vi "AOIParams.vi"() -> ()   [LabVIEW 2022 SP3]
uses:
  <vilib>/Utility/file.llb/Read Delimited Spreadsheet (DBL).vi
  <vilib>/Analysis/NI_AALBase.lvlib
panel:
  in  "Range Params":T1={"mb max"=-20.0, "mb min"=-70.0, "slope max"=8.0, "slope min"=-8.0, "int max"=5.0, "int min"=-85.0} {"int min" format="%.2f"; "int max" format="%.2f"; "slope min" format="%.2f"; "slope max" format="%.2f"; "mb min" format="%.2f"; "mb max" format="%.2f"}
  in  "data type":u16(ring)=1 items=["Spreadsheet", "byte file"]
  in  "Save to params.txt?":bool
  in  "Log scaling?":bool=TRUE
  out "mean of\nintercept":dbl format="%.3f"
  out "mean of\nslope":dbl format="%.3f"
  in  "Data for AOI":u16(ring)=2 items=["MidBand Fit Ellipse", "MidBand Fit Draw", "MidBand Fit Rect", "Slope Ellipse", "Slope Draw", "Slope Rect", "Intercept Ellipse", "Intercept Draw", "Intercept Rect"]
  out "RF Info":T2
  out "Array slope":dbl[][](array[numeric]) format="%.2f"
  out "Array midband":dbl[][](array[numeric]) format="%.2f"
  out "mean of\nmidband fit":dbl format="%.3f"
  in  "Use AOI":bool
  out "Array intercept":dbl[][](array[numeric]) format="%.2f"
  in  "Rotation":u32(knob) scale=0.18..180.0
  out "sector image":dbl[][](graph)
  out "raw eye data":i16[][](graph)
  out "Fit Param Image":dbl[][](graph)
  out "Fit band":T3 {"center freq" format="%.2f"; "stop freq" format="%.2f"; "start" format="%.2f"}
  in  "new eye file path":path
  # "Choose original eye file to run program. Parameter files must be in a sub-folder of the eye files named Param Images."
  # "© 2000 Riverside Research Institute"
  # "For ellipse use all three cursors, yellow is center. For free draw mode, yellow cursor will trace out aea. Start and stop free draw by pressing F1 key.For rectrangular mode, yellow and green form box. Yellow must be above and to left of green."
  # "(Ignore if Fit Param Image already in sector form)"
  # "Only needed for byte files"
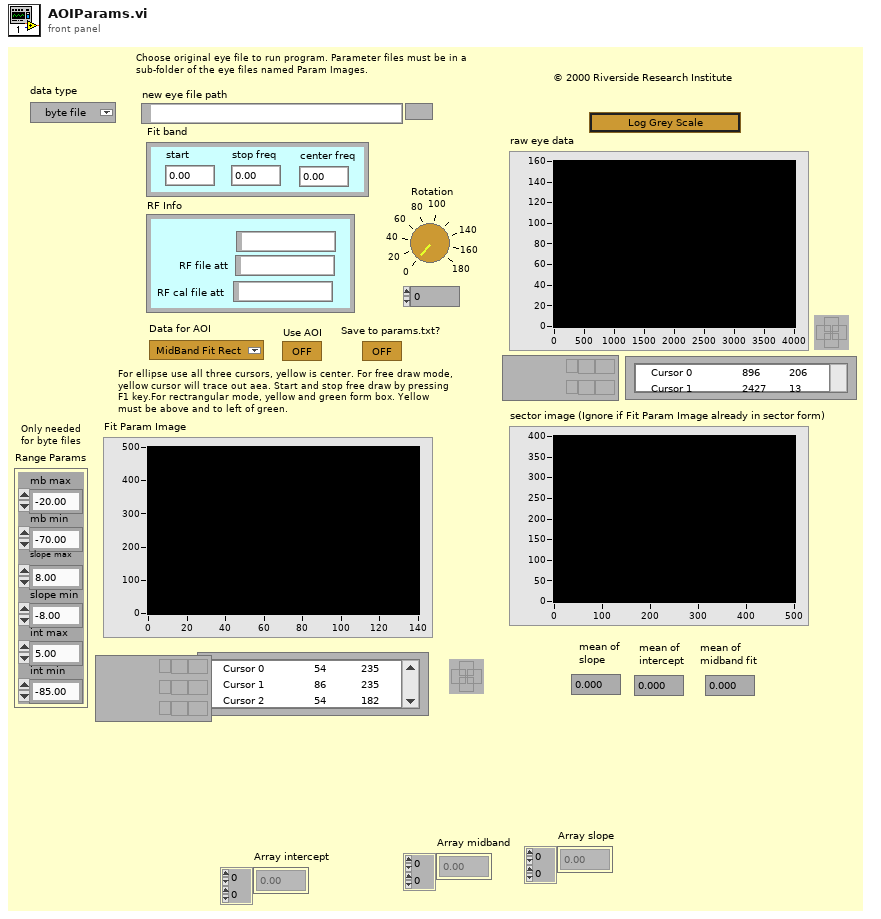
[diagram p1: front panel]
types:
  T1 = cluster{"mb max":dbl, "mb min":dbl, "slope max":dbl, "slope min":dbl, "int max":dbl, "int min":dbl}
  T2 = cluster{"RF file name":string, "RF file att":string, "RF cal file name":string, "RF cal file att":string}
  T3 = cluster{"start":dbl, "stop freq":dbl, "center freq":dbl}
  T4 = typedef "LVPointDoubleTypeDef.ctl" = cluster{"Cursor X":dbl, "Cursor Y":dbl}
  T5 = typedef "Header.ctl" = cluster{"header info":cluster{"Header":string, "Head length":i16}, "A/D info":cluster{"# rf points per line":u16, "# lines per scan":u16, "sample rate MHz":u16, "# A/D bits":i16, "# bytes per A/D":u16, "TGC Flag":u16, "A/D Type":string}, "Tranducer Info":cluster{"bandwidth":sgl, "center freq":sgl, "start freq":sgl, "ID":i32}, "Scan Info":cluster{"delay":sgl, "pivot distance":sgl, "sector scan angle":sgl, "operator":string, "Scan Mode":string, "location":string}, "Time/Date Info":cluster{"date":string, "time":string}, "RF Info":cluster{"RF file name":string, "RF file att":string, "RF cal file name":string, "RF cal file att":string}, "Patient Info":cluster{"ID":string, "extended ID":string, "age":u16, "sex":string, "previously\nscanned":string, "PSA":sgl, "LOS":u8, "Ethnicty 2":u8, "Race":u8}, "Tissue Type":cluster{"organ":i16, "disease type":i16, "disease location":i16, "IQ_pts":u16, "RcvBuffer":u8, "RcvFrame":u16, "IQBuff":u8, "IQFrame":u16, "IQPage":u8}, "Votage scaling":cluster{"Digitizer (dB)":sgl, "Gain (dB)":sgl, "Atten (dB)":sgl}, "Comment":string, "Misc Info":cluster{"avg num":u16, "c speed":i16, "Div By or SF zones":i16, "XMIT CHS":u8, "RCV CHS":u8, "Xmit angle":sgl}, "Therapy Parameters":cluster{"Theraputic Freq (MHz)":sgl, "Time on (s)":sgl, "Therapy amplitude (mV)":sgl, "Lines Before":u16, "Lines After":u16}, "Scan Settings":cluster{"Energy (uJ or V)":u8, "Damp (Ohm) or Fc":u8, "HP Filt (KHz)":u8, "LP Filt (MHz)":u8, "Gain (db)":u8, "prf (kHz)":sgl, "Distance between\nscan lines (um)":u16, "Distance between\nscan planes (um)":u16, "Scan line gap (um)":sgl, "Scan plane gap (um)":sgl}, "Compression Parameters":cluster{"F1 (MHz)":sgl, "F2 (MHz)":sgl, "% taper":sgl, "duration":sgl}, "Patient Info Xtra":cluster{"First Name":string, "Last Name":string, "Notes":string}, "ROI Box":u16[]}
  T6 = cluster{"delay":sgl, "pivot distance":sgl, "sector scan angle":sgl, "operator":string, "Scan Mode":string, "location":string}
  T7 = cluster{"start freq":sgl, sgl, "center freq":sgl}
  T8 = cluster{"Array Constant":dbl[], "Array Constant":dbl[]}
  T9 = cluster{"x start":i32, "length of x":i32, "y start":i32, "length of y":i32}
  T10 = cluster{"slope (m)":dbl, "intercept (b)":dbl, "midband fit":dbl, "pts in fit":dbl}
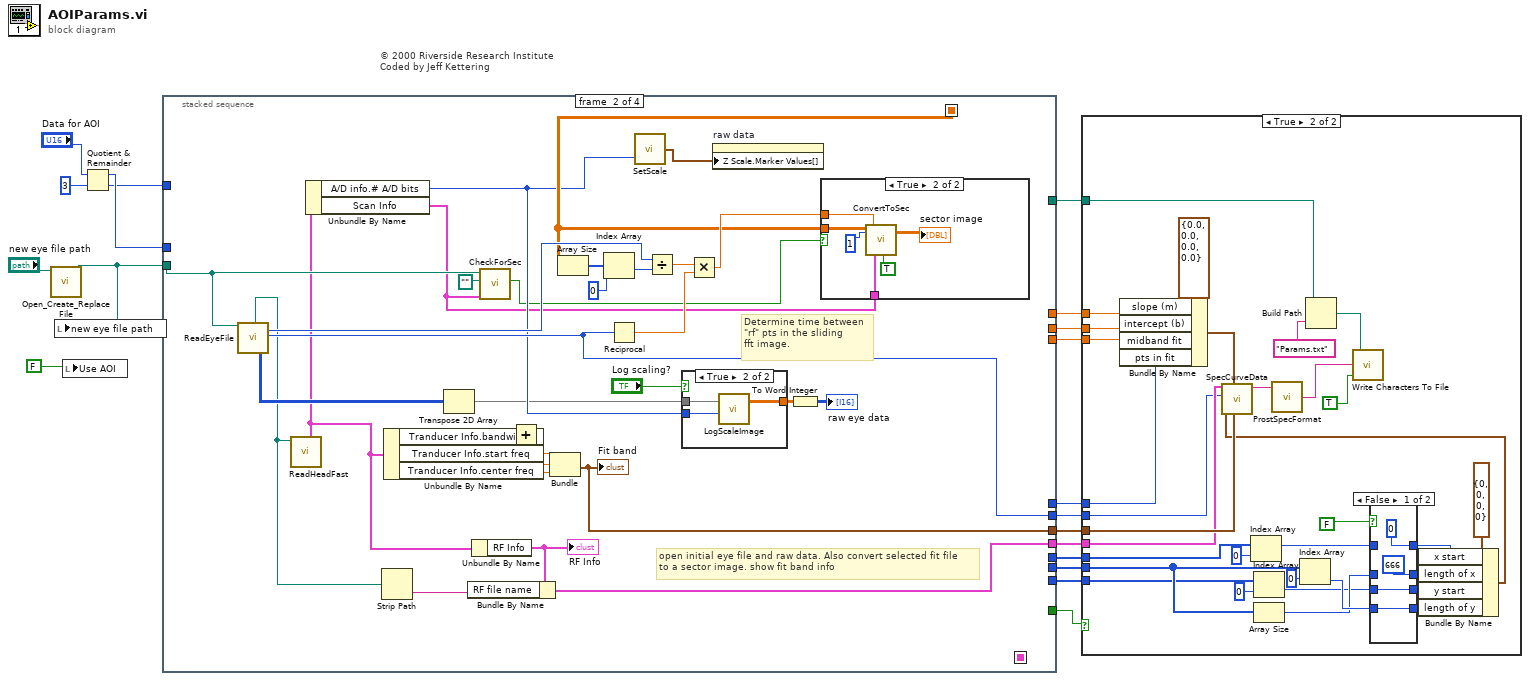
[diagram p0: block diagram]
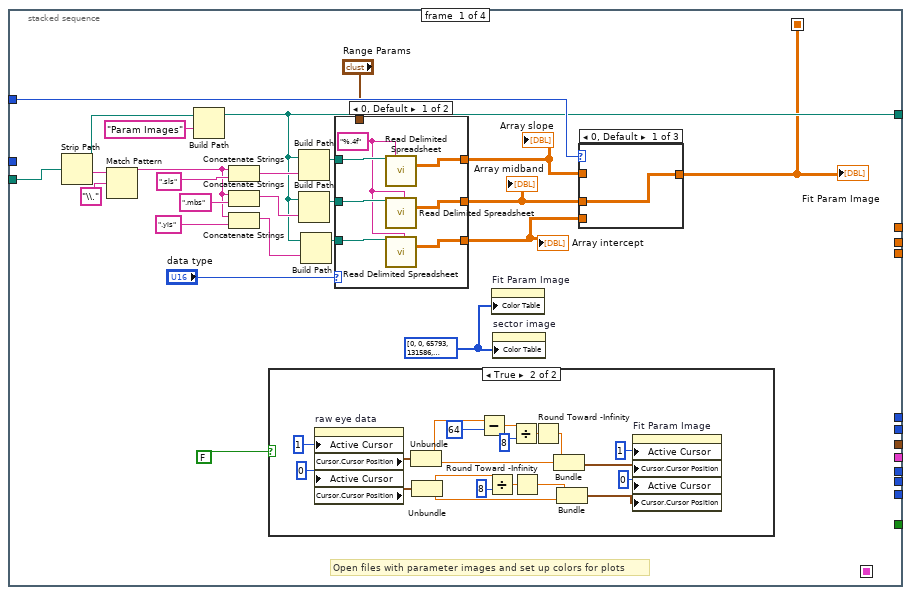
[diagram p4: hidden frame]
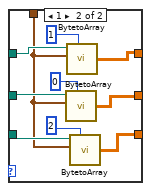
[diagram p5: hidden frame]
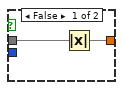
[diagram p10: hidden frame]
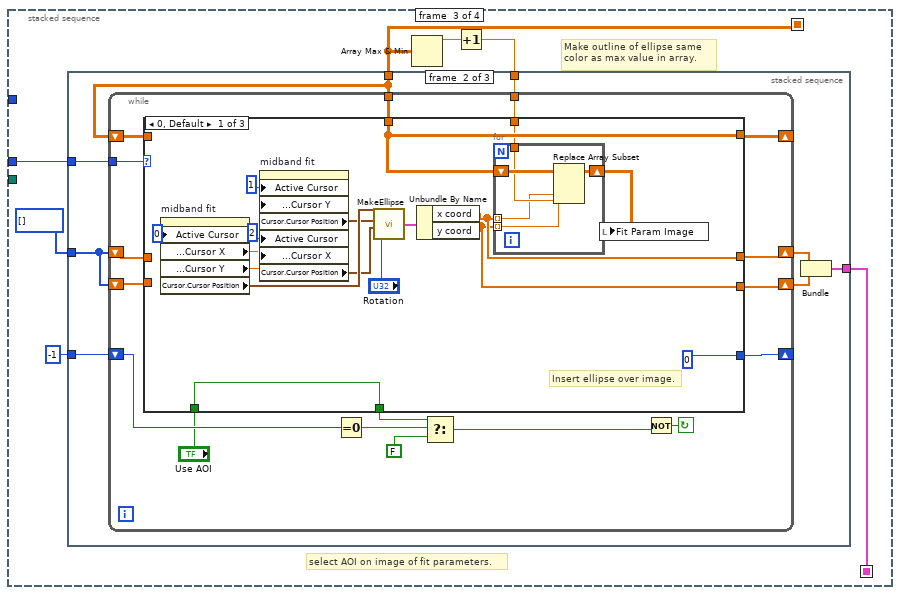
[diagram p11: hidden frame]
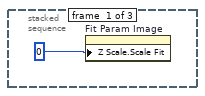
[diagram p12: hidden frame]
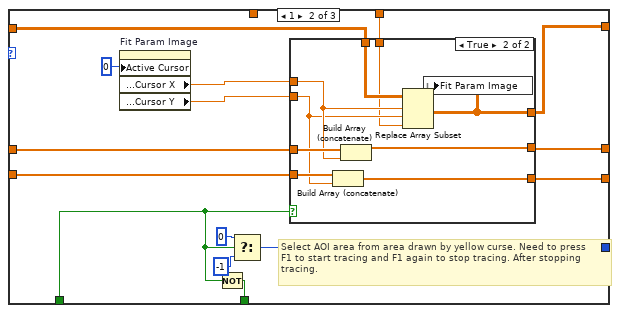
[diagram p13: hidden frame]
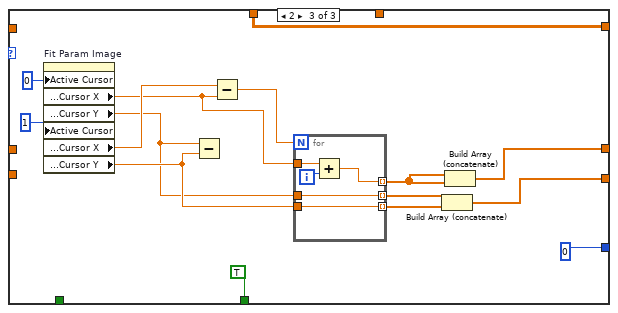
[diagram p15: hidden frame]
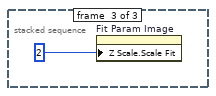
[diagram p16: hidden frame]
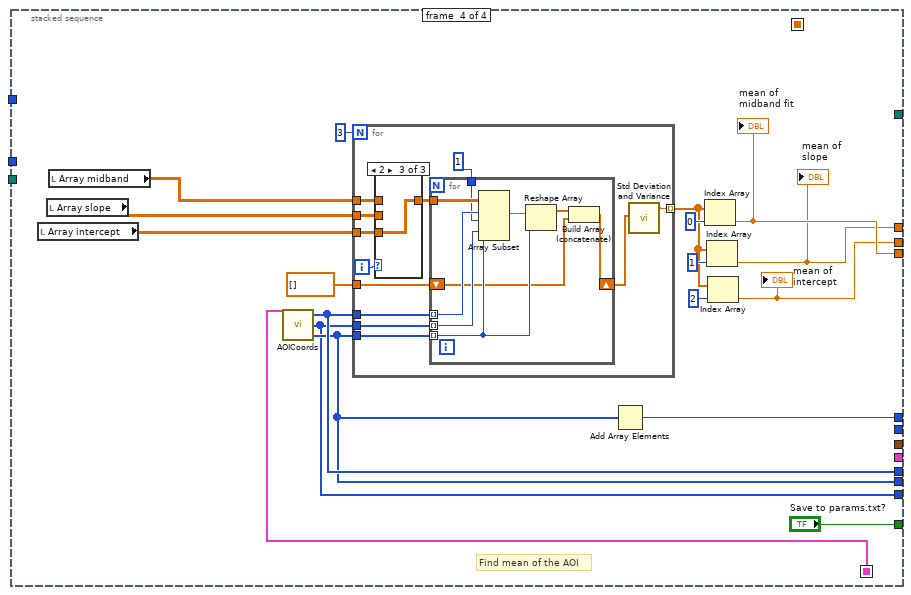
[diagram p17: hidden frame]
diagram:
  # "© 2000 Riverside Research Institute\nCoded by Jeff Kettering"
  n1 = call <vilib>:"Open_Create_Replace File.vi"("file path"="new eye file path") -> ("new file path"=w15:path)  [unwired: 5 in, 5 out]
  n2 = local write "new eye file path"(w15) -> ()
  n3 = local write "Use AOI"(FALSE) -> ()
  n4 = Quotient & Remainder(x="Data for AOI", y=u16 3) -> (x-y*floor(x/y)=w14:u16, floor(x/y)=w13:u16)
  n5 = stacked-sequence {
    seq-local: [_ _ w129 _] -> [_ _ _ w246]
    seq-local: [w20 _ _ _] -> [_ w101 w127 _]
    tunnel: w14 -> [_ _ w131 _]
    tunnel: w15 -> [w21 w95 _ _]
    tunnel: w13 -> [w29 _ _ _]
    tunnel: [_ _ _ w237] -> w10
    tunnel: [_ w97 _ _] -> w12
    tunnel: [w25 _ _ _] -> w11
    tunnel: [_ _ _ w235] -> w9
    tunnel: [_ _ _ w234] -> w8
    tunnel: [_ _ _ w233] -> w7
    tunnel: [_ w93 _ _] -> w6
    tunnel: [_ w96 _ _] -> w5
    tunnel: [_ _ _ "Save to params.txt?"] -> w4
    tunnel: [_ _ _ w231] -> w3
    tunnel: [_ _ _ w230] -> w2
    tunnel: [_ _ _ w229] -> w1
    frame #0 {
      w44 = u32[] [0, 0, 65793, 131586, 197379, 263172, 328965, 394758, 460551, 526344, 592137, 657930, 723723, 789516, 855309, 921102, 986895, 1052688, 1118481, 1184274, 1250067, 1315860, 1381653, 1447446, 1513239, 1579032, 1644825, 1710618, 1776411, 1842204, 1907997, 1973790, 2039583, 2105376, 2171169, 2236962, 2302755, 2368548, 2434341, 2500134, 2565927, 2631720, 2697513, 2763306, 2829099, 2894892, 2960685, 3026478, 3092271, 3158064, 3223857, 3289650, 3355443, 3421236, 3487029, 3552822, 3618615, 3684408, 3750201, 3815994, 3881787, 3947580, 4013373, 4079166, 4144959, 4210752, 4276545, 4342338, 4408131, 4473924, 4539717, 4605510, 4671303, 4737096, 4802889, 4868682, 4934475, 5000268, 5066061, 5131854, 5197647, 5263440, 5329233, 5395026, 5460819, 5526612, 5592405, 5658198, 5723991, 5789784, 5855577, 5921370, 5987163, 6052956, 6118749, 6184542, 6250335, 6316128, 6381921, 6447714, 6513507, 6579300, 6645093, 6710886, 6776679, 6842472, 6908265, 6974058, 7039851, 7105644, 7171437, 7237230, 7303023, 7368816, 7434609, 7500402, 7566195, 7631988, 7697781, 7763574, 7829367, 7895160, 7960953, 8026746, 8092539, 8158332, 8224125, 8289918, 8355711, 8421504, 8487297, 8553090, 8618883, 8684676, 8750469, 8816262, 8882055, 8947848, 9013641, 9079434, 9145227, 9211020, 9276813, 9342606, 9408399, 9474192, 9539985, 9605778, 9671571, 9737364, 9803157, 9868950, 9934743, 10000536, 10066329, 10132122, 10197915, 10263708, 10329501, 10395294, 10461087, 10526880, 10592673, 10658466, 10724259, 10790052, 10855845, 10921638, 10987431, 11053224, 11119017, 11184810, 11250603, 11316396, 11382189, 11447982, 11513775, 11579568, 11645361, 11711154, 11776947, 11842740, 11908533, 11974326, 12040119, 12105912, 12171705, 12237498, 12303291, 12369084, 12434877, 12500670, 12566463, 12632256, 12698049, 12763842, 12829635, 12895428, 12961221, 13027014, 13092807, 13158600, 13224393, 13290186, 13355979, 13421772, 13487565, 13553358, 13619151, 13684944, 13750737, 13816530, 13882323, 13948116, 14013909, 14079702, 14145495, 14211288, 14277081, 14342874, 14408667, 14474460, 14540253, 14606046, 14671839, 14737632, 14803425, 14869218, 14935011, 15000804, 15066597, 15132390, 15198183, 15263976, 15329769, 15395562, 15461355, 15527148, 15592941, 15658734, 15724527, 15790320, 15856113, 15921906, 15987699, 16053492, 16119285, 16185078, 16250871, 16316664, 16382457, 16448250, 16514043, 16579836, 16645629, 16711731] ("Read Attribute")
      # "Open files with parameter images and set up colors for plots"
      n6 = Strip Path(path=w21) -> (stripped path=w26:path, name=w32:string)
      n7 = Match Pattern(string=w32, regular expression="\\." ("search char (-)")) -> (before substring=w37:string)  [unwired: 4 out]
      n8 = Build Path(base path=w26, name or relative path="Param Images") -> (appended path=w25:path)
      n9 = Concatenate Strings(w37, ".sls") -> (w40:string)
      n10 = Concatenate Strings(w37, ".mbs") -> (w39:string)
      n11 = Concatenate Strings(w37, ".yis") -> (w38:string)
      n12 = case shown="True" FALSE ("Case Constant\n(See Context Help)") {
        frame False {
        }
        frame True {
          n13 = property on="raw eye data" class="IntGraph (strict)"("Active Cursor"=1, "Active Cursor"=0) -> ("Cursor.Cursor Position"=w76:T4, "Cursor.Cursor Position"=w77:T4)  [unwired: 2 in, 2 out]
          n14 = Unbundle(w76) -> ("Cursor X"=w67:dbl, "Cursor Y"=w72:dbl)
          n15 = Unbundle(w77) -> ("Cursor X"=w68:dbl, "Cursor Y"=w71:dbl)
          n16 = Subtract(x=w67, y=64) -> (x-y=w66:dbl)
          n17 = Divide(x=w68, y=8) -> (x/y=w70:dbl)
          n18 = Divide(x=w66, y=8) -> (x/y=w73:dbl)
          n19 = Round Toward -Infinity(1:w70) -> (0:w64:dbl)
          n20 = Round Toward -Infinity(1:w73) -> (0:w65:dbl)
          n21 = Bundle(w65, "Cursor Y"=w72) -> (w63:cluster{dbl, "Cursor Y":dbl})  [unwired: 1 out]
          n22 = Bundle(w64, "Cursor Y"=w71) -> (w62:cluster{dbl, "Cursor Y":dbl})  [unwired: 1 out]
          n23 = property on="Fit Param Image" class="IntGraph (strict)"("Active Cursor"=1, "Cursor.Cursor Position"=w63, "Active Cursor"=0, "Cursor.Cursor Position"=w62) -> ()  [unwired: 2 in, 2 out]
        }
      }
      n24 = Build Path(base path=w25, name or relative path=w40) -> (appended path=w36:path)
      n25 = Build Path(base path=w25, name or relative path=w39) -> (appended path=w35:path)
      n26 = Build Path(base path=w25, name or relative path=w38) -> (appended path=w34:path)
      n27 = case shown="0, Default" "data type" {
        tunnel: w36 -> [w51 w61]
        tunnel: w35 -> [w50 w59]
        tunnel: w34 -> [w49 w60]
        tunnel: [w47 w52] -> w24
        tunnel: [w46 w54] -> w31
        tunnel: [w45 w53] -> w30
        tunnel: "Range Params" -> [_ w58]
        frame 0, Default {
          w48 = "%.4f"
          n28 = call-poly <vilib>:"Read Delimited Spreadsheet.vi"("file path (dialog if empty)"=w51, "format (%.3f)"=w48) -> ("all rows"=w46:dbl[][])  [unwired: 8 in, 5 out]
          n29 = call-poly <vilib>:"Read Delimited Spreadsheet.vi"("file path (dialog if empty)"=w50, "format (%.3f)"=w48) -> ("all rows"=w45:dbl[][])  [unwired: 8 in, 5 out]
          n30 = call-poly <vilib>:"Read Delimited Spreadsheet.vi"("file path (dialog if empty)"=w49, "format (%.3f)"=w48) -> ("all rows"=w47:dbl[][])  [unwired: 8 in, 5 out]
        }
        frame 1 {
          n31 = call "BytetoArray.vi"("file path"=w59, "Ring"=0, "Range Params"=w58) -> ("Scaled data"=w53:dbl[][])  [unwired: 3 in, 2 out]
          n32 = call "BytetoArray.vi"("file path"=w61, "Ring"=1, "Range Params"=w58) -> ("Scaled data"=w54:dbl[][])  [unwired: 3 in, 2 out]
          n33 = call "BytetoArray.vi"("file path"=w60, "Ring"=2, "Range Params"=w58) -> ("Scaled data"=w52:dbl[][])  [unwired: 3 in, 2 out]
        }
      }
      "Array slope" <- w31
      "Array midband" <- w30
      "Array intercept" <- w24
      n34 = property on="Fit Param Image" class="IntGraph (strict)"("Color Table"=w44) -> ()  [unwired: 2 in, 2 out]
      n35 = property on="sector image" class="IntGraph (strict)"("Color Table"=w44) -> ()  [unwired: 2 in, 2 out]
      n36 = case shown="0, Default" w29 {
        tunnel: [w82 w83 w84] -> w20
        tunnel: w24 -> [_ _ w84]
        tunnel: w31 -> [_ w83 _]
        tunnel: w30 -> [w82 _ _]
        frame 0, Default {
        }
        frame 1 {
        }
        frame 2 {
        }
      }
      "Fit Param Image" <- w20
    }
    frame #1 {
      # "open initial eye file and raw data. Also convert selected fit file\nto a sector image. show fit band info"
      # "Determine time between\n\"rf\" pts in the sliding\nfft image."
      n37 = call "ReadEyeFile.vi"("new file path"=w95) -> ("new path out"=w89:path, "2-D data array"=w100:i16[][], "# rf points per line"=w114:u16, "sample rate MHz"=w96:u16)  [unwired: 1 in, 14 out]
      n38 = call "ReadHeadFast.vi"("new file path"=w89) -> ("Header In"=w86:T5)  [unwired: 7 in, 3 out]
      n39 = Unbundle By Name(w86) -> ("A/D info.# A/D bits"=w92:i16, "Scan Info"=w88:T6)
      n40 = Strip Path(path=w89) -> (name=w94:string)  [unwired: 1 out]
      n41 = Unbundle By Name(w86) -> ("Tranducer Info.bandwidth"=w105:sgl, "Tranducer Info.start freq"=w102:sgl, "Tranducer Info.center freq"=w104:sgl)
      n42 = Transpose 2D Array(2D array=w100) -> (transposed array=w90:i16[][])
      n43 = Unbundle By Name(w86) -> ("RF Info"=w85:T2)
      "RF Info" <- w85
      n44 = Bundle By Name(cluster=w85, "RF file name"=w94) -> (w93:T2)
      n45 = call "CheckForSec.vi"("Scan Info"=w88, "Last sector file opened"=path "", "Current file"=w95) -> ("sector?"=w87:bool)  [unwired: 6 out]
      n46 = Add(x=w105, y=w102) -> (x+y=w103:sgl)
      n47 = Bundle("start freq"=w102, w103, "center freq"=w104) -> (w97:T7)  [unwired: 1 out]
      "Fit band" <- w97
      n48 = Array Size(array=w101) -> (size(s)=w109:i32[])
      n49 = Index Array(array=w109, index=0 ("Index")) -> (element=w110:i32)
      n50 = Reciprocal(x=w96) -> (1/x=w112:dbl)
      n51 = call "SetScale.vi"("# A/D bits"=w92) -> ("Array"=w91:cluster{dbl, u32}[])  [unwired: 1 in]
      n52 = Divide(x=w114, y=w110) -> (x/y=w113:dbl)
      n53 = case shown="True" "Log scaling?" {
        tunnel: [w122 w125] -> w106
        tunnel: w90 -> [w121 w124]
        tunnel: w92 -> [_ w123]
        frame False {
          n54 = Absolute Value(x=w121) -> (abs(x)=w122:i16[][])
        }
        frame True {
          n55 = call "LogScaleImage.vi"("A/D bits"=w123, "input array"=w124) -> ("log scale image"=w125:dbl[][])  [unwired: 1 out]
        }
      }
      n56 = Multiply(x=w113, y=w112) -> (x*y=w111:dbl)
      n57 = property on="raw data" class="IntGraph (strict)"("Z Scale.Marker Values[]"=w91) -> ()  [unwired: 2 in, 2 out]
      n58 = To Word Integer(number=w106) -> (16bit integer=→"raw eye data":i16[][])
      n59 = case shown="True" w87 {
        tunnel: w111 -> [_ w120]
        tunnel: w88 -> [_ w117]
        tunnel: w101 -> [_ w116]
        frame False {
        }
        frame True {
          n60 = call "ConvertToSec.vi"("raw image data in"=w116, "reduce pts by factor of"=1, "Time between rf pts\nmicros"=w120, "Scan Info"=w117, "use min z value?"=TRUE) -> ("raw sector out"=→"sector image":dbl[][])  [unwired: 6 in, 8 out]
        }
      }
    }
    frame #2 {
      # "select AOI on image of fit parameters."
      # "Make outline of ellipse same \ncolor as max value in array."
      n61 = Array Max & Min(array=w127) -> (max value=w130:dbl)  [unwired: 3 out]
      n62 = Increment(x=w130) -> (x+1=w126:dbl)
      n63 = stacked-sequence {
        tunnel: i32[] [] ("Array Constant") -> [_ w134 _]
        tunnel: w131 -> [_ w141 _]
        tunnel: [_ w138 _] -> w129
        tunnel: -1 ("f") -> [_ w137 _]
        tunnel: w127 -> [_ w135 _]
        tunnel: w126 -> [_ w136 _]
        frame #0 {
          n64 = property on="Fit Param Image" class="IntGraph (strict)"("Z Scale.Scale Fit"=0) -> ()  [unwired: 2 in, 2 out]
        }
        frame #1 {
          n65 = while {
            shift-left: w137 -> [w147]
            shift-right: [w148] -> _
            tunnel: w136 -> [w149]
            tunnel: w141 -> [w150]
            shift-left: w135 -> [w151]
            shift-right: [w152] -> _
            shift-left: w134 -> [w155]
            shift-right: [w153] -> w139
            shift-left: w134 -> [w156]
            shift-right: [w154] -> w140
            tunnel: w135 -> [w157]
            stop <- w158 continue-if-true
            n66 = case shown="0, Default" w150 {
              tunnel: w157 -> [w165 _ w218]
              tunnel: w156 -> [_ w195 _]
              tunnel: w155 -> [_ w194 _]
              tunnel: [w163 w193 w210] -> w154
              tunnel: [w162 w192 w209] -> w153
              tunnel: [w165 w190 w218] -> w152
              tunnel: w151 -> [_ w191 _]
              tunnel: w149 -> [w164 w189 _]
              tunnel: [0 w188 0] -> w148
              tunnel: [w159 w187 TRUE] -> w143
              tunnel: "Use AOI" -> [w159 w181 _]
              frame 0, Default {
                # "Insert ellipse over image."
                n67 = property on="midband fit" class="IntGraph (strict)"("Active Cursor"=u32 0 ("Write Attribute")) -> ("Cursor.Cursor Position:Cursor X"=w170:dbl, "Cursor.Cursor Position:Cursor Y"=w171:dbl, "Cursor.Cursor Position"=w169:T4)  [unwired: 2 in, 2 out]
                n68 = property on="midband fit" class="IntGraph (strict)"("Active Cursor"=u32 1 ("Write Attribute"), "Cursor.Cursor Position:Cursor Y"=w171, "Active Cursor"=u32 2 ("Write Attribute"), "Cursor.Cursor Position:Cursor X"=w170) -> ("Cursor.Cursor Position"=w168:T4, "Cursor.Cursor Position"=w167:T4)  [unwired: 2 in, 2 out]
                n69 = call "MakeEllipse.vi"("Rotation"="Rotation", "Cursor 2"=w167, "Cursor 1"=w168, "Cursor 0"=w169) -> ("X-Y elipse"=w175:cluster{"x coord":dbl[], "y coord":dbl[]})
                n70 = Unbundle By Name(w175) -> ("x coord"=w163:dbl[], "y coord"=w162:dbl[])
                n71 = for {
                  tunnel: w163 -> [w177] mode=indexing
                  tunnel: w162 -> [w176] mode=indexing
                  shift-right: [w179] -> w160
                  shift-left: w165 -> [w180]
                  tunnel: w164 -> [w178]
                  n72 = Replace Array Subset(array=w180, new element=w178, index (row)=w177, index (col)=w176) -> (w179:dbl[][])
                }
                n73 = local write "Fit Param Image"(w160) -> ()
              }
              frame 1 {
                # "Select AOI area from area drawn by yellow curse. Need to press\nF1 to start tracing and F1 again to stop tracing. After stopping\ntracing."
                n74 = property on="Fit Param Image" class="IntGraph (strict)"("Active Cursor"=u32 0 ("Write Attribute")) -> ("Cursor.Cursor Position:Cursor X"=w186:dbl, "Cursor.Cursor Position:Cursor Y"=w185:dbl)  [unwired: 2 in, 2 out]
                n75 = Not(x=w181) -> (.not. x?=w187:bool)
                n76 = Select(t=0, s=w181, f=-1) -> (s? t:f=w188:i32)
                n77 = case shown="True" w181 {
                  tunnel: w194 -> [w197 w207]
                  tunnel: [w197 w206] -> w192
                  tunnel: [w198 w205] -> w193
                  tunnel: w195 -> [w198 w204]
                  tunnel: w186 -> [_ w203]
                  tunnel: w185 -> [_ w202]
                  tunnel: [w196 w199] -> w190
                  tunnel: w191 -> [w196 w201]
                  tunnel: w189 -> [_ w200]
                  frame False {
                  }
                  frame True {
                    n78 = Build Array (concatenate)(w207, w202) -> (w206:dbl[])
                    n79 = Build Array (concatenate)(w204, w203) -> (w205:dbl[])
                    n80 = Replace Array Subset(array=w201, new element=w200, index (row)=w203, index (col)=w202) -> (w199:dbl[][])
                    n81 = local write "Fit Param Image"(w199) -> ()
                  }
                }
              }
              frame 2 {
                n82 = property on="Fit Param Image" class="IntGraph (strict)"("Active Cursor"=0, "Active Cursor"=1) -> ("Cursor.Cursor Position:Cursor X"=w216:dbl, "Cursor.Cursor Position:Cursor Y"=w214:dbl, "Cursor.Cursor Position:Cursor X"=w220:dbl, "Cursor.Cursor Position:Cursor Y"=w215:dbl)  [unwired: 2 in, 2 out]
                n83 = Subtract(x=w214, y=w215) -> ()  [unwired: 1 out]
                n84 = Subtract(x=w220, y=w216) -> (x-y=w217:dbl)
                n85 = for {
                  N: w217 -> [_]
                  tunnel: w216 -> [w227]
                  tunnel: [w225] -> w211 mode=indexing
                  tunnel: w215 -> [w225]
                  tunnel: w214 -> [w223]
                  tunnel: [w224] -> w213 mode=indexing
                  tunnel: [w223] -> w212 mode=indexing
                  i -> [w226]
                  n86 = Add(x=w227, y=w226) -> (x+y=w224:dbl)
                }
                n87 = Build Array (concatenate)(w212, w211) -> (w209:dbl[])
                n88 = Build Array (concatenate)(w213, w213) -> (w210:dbl[])
              }
            }
            n89 = Equal To 0?(x=w147) -> (x = 0?=w146:bool)
            n90 = Select(t=w143, s=w146, f=FALSE) -> (s? t:f=w145:bool)
            n91 = Not(x=w145) -> (.not. x?=w158:bool)
          }
          n92 = Bundle("Array Constant"=w140, "Array Constant"=w139) -> (w138:T8)  [unwired: 1 out]
        }
        frame #2 {
          n93 = property on="Fit Param Image" class="IntGraph (strict)"("Z Scale.Scale Fit"=2) -> ()  [unwired: 2 in, 2 out]
        }
      }
    }
    frame #3 {
      # "Find mean of the AOI"
      n94 = local read "Array intercept"() -> (w241:dbl[][])
      n95 = local read "Array slope"() -> (w240:dbl[][])
      n96 = local read "Array midband"() -> (w239:dbl[][])
      n97 = call "AOICoords.vi"("X-Y data"=w246) -> ("start row for pts"=w231:i32[], "start column for pts"=w229:i32[], "# pts to take in row"=w230:i32[])  [unwired: 4 out]
      n98 = for {
        N: 3 -> [_]
        tunnel: w230 -> [w257]
        tunnel: w229 -> [w256]
        tunnel: w231 -> [w255]
        tunnel: w239 -> [w253]
        tunnel: w240 -> [w251]
        tunnel: w241 -> [w250]
        tunnel: [w249] -> w238 mode=indexing
        tunnel: dbl[] [] ("Array Constant") -> [w248]
        i -> [w254]
        n99 = case shown="2" w254 {
          tunnel: [w259 w260 w261] -> w252
          tunnel: w253 -> [w259 _ _]
          tunnel: w251 -> [_ w260 _]
          tunnel: w250 -> [_ _ w261]
          frame 0, Default {
          }
          frame 1 {
          }
          frame 2 {
          }
        }
        n100 = for {
          tunnel: w255 -> [w269] mode=indexing
          tunnel: w256 -> [w268] mode=indexing
          tunnel: w257 -> [w266] mode=indexing
          tunnel: w252 -> [w270]
          tunnel: 1 -> [w267]
          shift-right: [w263] -> w247
          shift-left: w248 -> [w262]
          n101 = Array Subset(array=w270, index (row)=w269, length (row)=w267, index (col)=w268, length (col)=w266) -> (w265:dbl[][])
          n102 = Reshape Array(w265, w266) -> (w264:dbl[])
          n103 = Build Array (concatenate)(w264, w262) -> (w263:dbl[])
        }
        n104 = call <vilib>:"Std Deviation and Variance.vi"("X"=w247) -> ("mean"=w249:dbl)  [unwired: 1 in, 2 out]
      }
      n105 = Add Array Elements(numeric array=w230) -> (sum=w237:i32)
      n106 = Index Array(array=w238, index=0 ("Index")) -> (element=w235:dbl)
      "mean of\nmidband fit" <- w235
      n107 = Index Array(array=w238, index=1 ("Index")) -> (element=w233:dbl)
      "mean of\nslope" <- w233
      n108 = Index Array(array=w238, index=2 ("Index")) -> (element=w234:dbl)
      "mean of\nintercept" <- w234
    }
  }
  n109 = case shown="True" w4 {
    tunnel: w12 -> [_ w298]
    tunnel: w11 -> [_ w282]
    tunnel: w10 -> [_ w296]
    tunnel: w9 -> [_ w283]
    tunnel: w8 -> [_ w295]
    tunnel: w7 -> [_ w294]
    tunnel: w6 -> [_ w293]
    tunnel: w5 -> [_ w292]
    tunnel: w3 -> [_ w288]
    tunnel: w2 -> [_ w287]
    tunnel: w1 -> [_ w286]
    frame False {
    }
    frame True {
      n110 = Bundle By Name(cluster=T10 {"slope (m)"=0.0, "intercept (b)"=0.0, "midband fit"=0.0, "pts in fit"=0.0} ("Fit params"), "slope (m)"=w294, "intercept (b)"=w295, "midband fit"=w283, "pts in fit"=w296) -> (w299:T10)
      n111 = Index Array(array=w288, index=0 ("Index")) -> (element=w281:i32)
      n112 = Index Array(array=w286, index=0 ("Index")) -> (element=w278:i32)
      n113 = Array Size(array=w287) -> (size(s)=w279:i32)
      n114 = Index Array(array=w287, index=0 ("Index")) -> (element=w280:i32)
      n115 = Build Path(base path=w282, name or relative path="Params.txt") -> (appended path=w297:path)
      n116 = case shown="False" FALSE ("Case Constant\n(See Context Help) 2") {
        tunnel: [0 w310] -> w277
        tunnel: w281 -> [_ w310]
        tunnel: [w306 w309] -> w274
        tunnel: w280 -> [w306 w309]
        tunnel: [w305 w308] -> w275
        tunnel: w278 -> [w305 w308]
        tunnel: [666 w307] -> w276
        tunnel: w279 -> [_ w307]
        frame False {
        }
        frame True {
        }
      }
      n117 = Bundle By Name(cluster=T9 {"x start"=0, "length of x"=0, "y start"=0, "length of y"=0} ("Array Subset"), "x start"=w277, "length of x"=w276, "y start"=w275, "length of y"=w274) -> (w285:T9)
      n118 = call "SpecCurveData.vi"("Fit band"=w298, "Fit params"=w299, "Array Subset"=w285, "sample rate MHz"=w292, "RF Info"=w293) -> ("Spectra data"=w272:string)  [unwired: 2 in, 4 out]
      n119 = call "ProstSpecFormat.vi"("Spectra.txt old (string)"=w272) -> ("Spectra.txt new out"=w271:string)
      n120 = call <vilib>:"Write Characters To File.vi"("append to file? (new file:F)"=TRUE, "character string"=w271, "file path (dialog if empty)"=w297) -> ()  [unwired: 3 out]
    }
  }
